vi "Elapsed Time String.vi"() -> (0 "Elapsed Time":string)   [LabVIEW 2019, in "Instrument UI.PPMS.lvclass"]
uses:
  Instrument UI.PPMS.lvclass
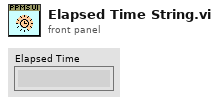
[diagram p1: front panel]
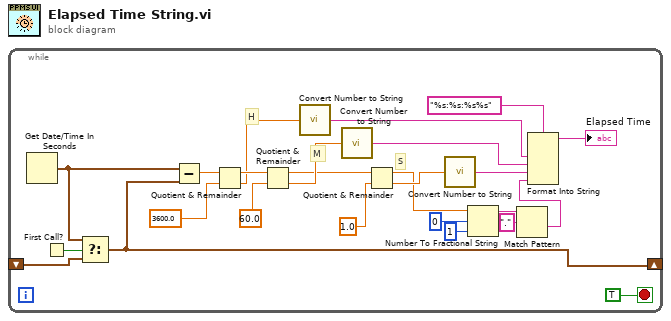
[diagram p0: block diagram]
diagram:
  n1 = while {
    shift-right: [w16] -> _
    shift-left: _ -> [w18]
    stop <- TRUE stop-if-true
    # "S"
    # "M"
    # "H"
    n2 = Get Date/Time In Seconds() -> (seconds since 1Jan1904=w17:timestamp)
    n3 = First Call?() -> (First Call?: T/F=w19:bool)
    n4 = Select(t=w17, s=w19, f=w18) -> (s? t:f=w16:timestamp)
    n5 = Subtract(x=w17, y=w16) -> (x-y=w20:dbl)
    n6 = Quotient & Remainder(x=w20, y=3600.0) -> (x-y*floor(x/y)=w24:dbl, floor(x/y)=w13:dbl)
    n7 = Quotient & Remainder(x=w24, y=60.0) -> (x-y*floor(x/y)=w8:dbl, floor(x/y)=w12:dbl)
    n8 = call "Convert Number to String.vi"("Numeric"=w13) -> ("String"=w14:string)
    n9 = call "Convert Number to String.vi"("Numeric"=w12) -> ("String"=w11:string)
    n10 = Quotient & Remainder(x=w8, y=1.0) -> (x-y*floor(x/y)=w1:dbl, floor(x/y)=w7:dbl)
    n11 = call "Convert Number to String.vi"("Numeric"=w7) -> ("String"=w9:string)
    n12 = Number To Fractional String(number=w1, width (-)=i16 0, precision (6)=i16 1 ("width (-)")) -> (F-format string=w3:string)  [unwired: 1 in]
    n13 = Match Pattern(string=w3, regular expression=".") -> (after substring=w2:string)  [unwired: 1 in, 3 out]
    n14 = Format Into String(format string="%s:%s:%s%s", w14, w11, w9, w2) -> (resulting string=→"Elapsed Time":string)  [unwired: 2 in, 1 out]
  }
